vi "DAQmx Get Channel Property (CI Frequency Measurement Time).vi"(0 "task in":refnum<class "Session Factory.lvclass">, 11 "error in":errorcluster) -> (4 "task out":refnum<class "Session Factory.lvclass">, 6 "CI.Freq.MeasTime":dbl, 15 "error out":errorcluster)   [LabVIEW 2021, in "Session Management niDAQmx.lvlib" / "Session Factory.lvclass"]
doc: "<B>Property: Get DAQmx Channel (Counter Input:Frequency:Measurement Specifications:High Frequency:Measurement Time)</B>\n\nShort Name: <B>CI.Freq.MeasTime</B>\n\nSpecifies in seconds the length of time to measure the frequency of the signal if CI.Freq.MeasMeth is High Frequency with 2 Counters. Measurement accuracy increases with increased measurement time and with increased signal frequency. If you measure a high-frequency signal for too long, however, the count register could roll over, which results in an incorrect measurement."
uses:
  Session Factory.lvclass
  NI_DAQmx_client/RPC Messages/nidaqmx_grpc_GetChanAttributeDoubleRequest.ctl
  NI_DAQmx_client/RPC Messages/nidevice_grpc_Session.ctl
  NI_DAQmx_client/RPC Messages/nidevice_grpc_Session_session/nidevice_grpc_Session_session.lvclass
  NI_DAQmx_client/RPC Messages/nidaqmx_grpc_GetChanAttributeDoubleRequest_attribute_enum/nidaqmx_grpc_GetChanAttributeDoubleRequest_attribute_enum.lvclass
  NI_DAQmx_client/RPC Messages/nidaqmx_grpc_ChannelDoubleAttribute.ctl
  NI_DAQmx_client/RPC Messages/nidaqmx_grpc_GetChanAttributeDoubleRequest_attribute_enum/nidaqmx_grpc_GetChanAttributeDoubleRequest_attribute_enum.lvclass/nidaqmx_grpc_GetChanAttributeDoubleRequest_attribute_enum.ctl
  Session Factory.lvclass/Session Factory.ctl
  NI_DAQmx_client/NI_DAQmx_client.lvlib
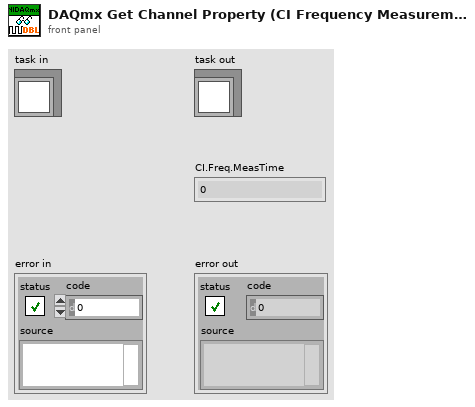
[diagram p1: front panel]
types:
  T1 = typedef "NI_DAQmx_client.lvlib/nidaqmx_grpc_ChannelDoubleAttribute.ctl" = enum32{"CHANNEL_DOUBLE_ATTRIBUTE_UNSPECIFIED", "CHANNEL_ATTRIBUTE_AI_IMPEDANCE", "CHANNEL_ATTRIBUTE_AI_AC_EXCIT_FREQ", "CHANNEL_ATTRIBUTE_AO_GAIN", "CHANNEL_ATTRIBUTE_AO_LOAD_IMPEDANCE", "CHANNEL_ATTRIBUTE_CI_FREQ_MEAS_TIME", "CHANNEL_ATTRIBUTE_CO_PULSE_FREQ_INITIAL_DELAY", "CHANNEL_ATTRIBUTE_AI_ACCEL_SENSITIVITY", "CHANNEL_ATTRIBUTE_AI_FREQ_HYST", "CHANNEL_ATTRIBUTE_AI_FREQ_THRESH_VOLTAGE", "CHANNEL_ATTRIBUTE_CI_ANG_ENCODER_INITIAL_ANGLE", "CHANNEL_ATTRIBUTE_CI_ENCODER_Z_INDEX_VAL", "CHANNEL_ATTRIBUTE_AI_RVDT_SENSITIVITY", "CHANNEL_ATTRIBUTE_CI_LIN_ENCODER_DIST_PER_PULSE", "CHANNEL_ATTRIBUTE_CI_LIN_ENCODER_INITIAL_POS", "CHANNEL_ATTRIBUTE_AI_LVDT_SENSITIVITY", "CHANNEL_ATTRIBUTE_AI_STRAIN_GAGE_GAGE_FACTOR", "CHANNEL_ATTRIBUTE_AI_STRAIN_GAGE_POISSON_RATIO", "CHANNEL_ATTRIBUTE_AI_RTD_A", "CHANNEL_ATTRIBUTE_AI_RTD_B", "CHANNEL_ATTRIBUTE_AI_RTD_C", "CHANNEL_ATTRIBUTE_AI_RTD_R0", "CHANNEL_ATTRIBUTE_AI_THRMCPL_CJC_VAL", "CHANNEL_ATTRIBUTE_AI_THRMSTR_R1", "CHANNEL_ATTRIBUTE_CO_PULSE_DUTY_CYC", "CHANNEL_ATTRIBUTE_CO_PULSE_FREQ", "CHANNEL_ATTRIBUTE_AO_MAX", "CHANNEL_ATTRIBUTE_AO_MIN", "CHANNEL_ATTRIBUTE_AO_OUTPUT_IMPEDANCE", "CHANNEL_ATTRIBUTE_AI_MICROPHONE_SENSITIVITY", "CHANNEL_ATTRIBUTE_AI_RESOLUTION", "CHANNEL_ATTRIBUTE_AI_MAX", "CHANNEL_ATTRIBUTE_AI_MIN", "CHANNEL_ATTRIBUTE_AI_BRIDGE_NOM_RESISTANCE", "CHANNEL_ATTRIBUTE_AI_BRIDGE_INITIAL_VOLTAGE", "CHANNEL_ATTRIBUTE_AI_LEAD_WIRE_RESISTANCE", "CHANNEL_ATTRIBUTE_AI_CURRENT_SHUNT_RESISTANCE", "CHANNEL_ATTRIBUTE_AI_EXCIT_VAL", "CHANNEL_ATTRIBUTE_AI_ATTEN", "CHANNEL_ATTRIBUTE_AI_LOWPASS_CUTOFF_FREQ", "CHANNEL_ATTRIBUTE_AI_HIGHPASS_CUTOFF_FREQ", "CHANNEL_ATTRIBUTE_AI_BANDPASS_CENTER_FREQ", "CHANNEL_ATTRIBUTE_AI_BANDPASS_WIDTH", "CHANNEL_ATTRIBUTE_AI_NOTCH_CENTER_FREQ", "CHANNEL_ATTRIBUTE_AI_NOTCH_WIDTH", "CHANNEL_ATTRIBUTE_AI_RNG_HIGH", "CHANNEL_ATTRIBUTE_AI_RNG_LOW", "CHANNEL_ATTRIBUTE_AI_GAIN", "CHANNEL_ATTRIBUTE_AO_RESOLUTION", "CHANNEL_ATTRIBUTE_AO_DAC_RNG_LOW", "CHANNEL_ATTRIBUTE_AO_DAC_RNG_HIGH", "CHANNEL_ATTRIBUTE_AO_DAC_REF_VAL", "CHANNEL_ATTRIBUTE_AI_EXCIT_ACTUAL_VAL", "CHANNEL_ATTRIBUTE_AI_LOWPASS_SWITCH_CAP_EXT_CLK_FREQ", "CHANNEL_ATTRIBUTE_CI_MAX", "CHANNEL_ATTRIBUTE_CI_MIN", "CHANNEL_ATTRIBUTE_CI_CTR_TIMEBASE_RATE", "CHANNEL_ATTRIBUTE_CO_PULSE_HIGH_TIME", "CHANNEL_ATTRIBUTE_CO_PULSE_LOW_TIME", "CHANNEL_ATTRIBUTE_CO_PULSE_TIME_INITIAL_DELAY", "CHANNEL_ATTRIBUTE_CO_CTR_TIMEBASE_RATE", "CHANNEL_ATTRIBUTE_AI_THRMSTR_A", "CHANNEL_ATTRIBUTE_AI_THRMSTR_C", "CHANNEL_ATTRIBUTE_AI_THRMSTR_B", "CHANNEL_ATTRIBUTE_CI_PERIOD_MEAS_TIME", "CHANNEL_ATTRIBUTE_AI_BRIDGE_SHUNT_CAL_GAIN_ADJUST", "CHANNEL_ATTRIBUTE_DI_DIG_FLTR_MIN_PULSE_WIDTH", "CHANNEL_ATTRIBUTE_CI_FREQ_DIG_FLTR_MIN_PULSE_WIDTH", "CHANNEL_ATTRIBUTE_CI_FREQ_DIG_FLTR_TIMEBASE_RATE", "CHANNEL_ATTRIBUTE_CI_PERIOD_DIG_FLTR_MIN_PULSE_WIDTH", "CHANNEL_ATTRIBUTE_CI_PERIOD_DIG_FLTR_TIMEBASE_RATE", "CHANNEL_ATTRIBUTE_CI_COUNT_EDGES_COUNT_DIR_DIG_FLTR_MIN_PULSE_WIDTH", "CHANNEL_ATTRIBUTE_CI_COUNT_EDGES_COUNT_DIR_DIG_FLTR_TIMEBASE_RATE", "CHANNEL_ATTRIBUTE_CI_COUNT_EDGES_DIG_FLTR_MIN_PULSE_WIDTH", "CHANNEL_ATTRIBUTE_CI_COUNT_EDGES_DIG_FLTR_TIMEBASE_RATE", "CHANNEL_ATTRIBUTE_CI_ENCODER_A_INPUT_DIG_FLTR_MIN_PULSE_WIDTH", "CHANNEL_ATTRIBUTE_CI_ENCODER_A_INPUT_DIG_FLTR_TIMEBASE_RATE", "CHANNEL_ATTRIBUTE_CI_ENCODER_B_INPUT_DIG_FLTR_MIN_PULSE_WIDTH", "CHANNEL_ATTRIBUTE_CI_ENCODER_B_INPUT_DIG_FLTR_TIMEBASE_RATE", "CHANNEL_ATTRIBUTE_CI_ENCODER_Z_INPUT_DIG_FLTR_MIN_PULSE_WIDTH", "CHANNEL_ATTRIBUTE_CI_ENCODER_Z_INPUT_DIG_FLTR_TIMEBASE_RATE", "CHANNEL_ATTRIBUTE_CI_PULSE_WIDTH_DIG_FLTR_MIN_PULSE_WIDTH", "CHANNEL_ATTRIBUTE_CI_PULSE_WIDTH_DIG_FLTR_TIMEBASE_RATE", "CHANNEL_ATTRIBUTE_CI_TWO_EDGE_SEP_FIRST_DIG_FLTR_MIN_PULSE_WIDTH", "CHANNEL_ATTRIBUTE_CI_TWO_EDGE_SEP_FIRST_DIG_FLTR_TIMEBASE_RATE", "CHANNEL_ATTRIBUTE_CI_TWO_EDGE_SEP_SECOND_DIG_FLTR_MIN_PULSE_WIDTH", "CHANNEL_ATTRIBUTE_CI_TWO_EDGE_SEP_SECOND_DIG_FLTR_TIMEBASE_RATE", "CHANNEL_ATTRIBUTE_CI_SEMI_PERIOD_DIG_FLTR_MIN_PULSE_WIDTH", "CHANNEL_ATTRIBUTE_CI_SEMI_PERIOD_DIG_FLTR_TIMEBASE_RATE", "CHANNEL_ATTRIBUTE_AI_SOUND_PRESSURE_MAX_SOUND_PRESSURE_LVL", "CHANNEL_ATTRIBUTE_AO_DAC_OFFSET_VAL", "CHANNEL_ATTRIBUTE_CI_CTR_TIMEBASE_DIG_FLTR_MIN_PULSE_WIDTH", "CHANNEL_ATTRIBUTE_CI_CTR_TIMEBASE_DIG_FLTR_TIMEBASE_RATE", "CHANNEL_ATTRIBUTE_CO_CTR_TIMEBASE_DIG_FLTR_MIN_PULSE_WIDTH", "CHANNEL_ATTRIBUTE_CO_CTR_TIMEBASE_DIG_FLTR_TIMEBASE_RATE", "CHANNEL_ATTRIBUTE_AI_VOLTAGE_DB_REF", "CHANNEL_ATTRIBUTE_AI_SOUND_PRESSURE_DB_REF", "CHANNEL_ATTRIBUTE_AI_ACCEL_DB_REF", "CHANNEL_ATTRIBUTE_AO_FUNC_GEN_FREQ", "CHANNEL_ATTRIBUTE_AO_FUNC_GEN_AMPLITUDE", "CHANNEL_ATTRIBUTE_AO_FUNC_GEN_OFFSET", "CHANNEL_ATTRIBUTE_AO_FUNC_GEN_SQUARE_DUTY_CYCLE", "CHANNEL_ATTRIBUTE_AO_VOLTAGE_CURRENT_LIMIT", "CHANNEL_ATTRIBUTE_AO_FUNC_GEN_FM_DEVIATION", "CHANNEL_ATTRIBUTE_DO_OVERCURRENT_LIMIT", "CHANNEL_ATTRIBUTE_DO_OVERCURRENT_REENABLE_PERIOD", "CHANNEL_ATTRIBUTE_AI_PROBE_ATTEN", "CHANNEL_ATTRIBUTE_AI_DC_OFFSET", "CHANNEL_ATTRIBUTE_AI_EDDY_CURRENT_PROX_PROBE_SENSITIVITY", "CHANNEL_ATTRIBUTE_DI_DIG_FLTR_TIMEBASE_RATE", "CHANNEL_ATTRIBUTE_CI_PULSE_FREQ_DIG_FLTR_MIN_PULSE_WIDTH", "CHANNEL_ATTRIBUTE_CI_PULSE_FREQ_DIG_FLTR_TIMEBASE_RATE", "CHANNEL_ATTRIBUTE_CI_PULSE_TIME_DIG_FLTR_MIN_PULSE_WIDTH", "CHANNEL_ATTRIBUTE_CI_PULSE_TIME_DIG_FLTR_TIMEBASE_RATE", "CHANNEL_ATTRIBUTE_CI_PULSE_TICKS_DIG_FLTR_MIN_PULSE_WIDTH", "CHANNEL_ATTRIBUTE_CI_PULSE_TICKS_DIG_FLTR_TIMEBASE_RATE", "CHANNEL_ATTRIBUTE_AI_BRIDGE_SHUNT_CAL_SHUNT_CAL_A_RESISTANCE", "CHANNEL_ATTRIBUTE_AI_BRIDGE_SHUNT_CAL_SHUNT_CAL_A_ACTUAL_RESISTANCE", "CHANNEL_ATTRIBUTE_AI_BRIDGE_SHUNT_CAL_SHUNT_CAL_B_RESISTANCE", "CHANNEL_ATTRIBUTE_AI_BRIDGE_SHUNT_CAL_SHUNT_CAL_B_ACTUAL_RESISTANCE", "CHANNEL_ATTRIBUTE_AI_FORCE_IEPE_SENSOR_SENSITIVITY", "CHANNEL_ATTRIBUTE_AI_BRIDGE_INITIAL_RATIO", "CHANNEL_ATTRIBUTE_AI_BRIDGE_TWO_POINT_LIN_FIRST_ELECTRICAL_VAL", "CHANNEL_ATTRIBUTE_AI_BRIDGE_TWO_POINT_LIN_FIRST_PHYSICAL_VAL", "CHANNEL_ATTRIBUTE_AI_BRIDGE_TWO_POINT_LIN_SECOND_ELECTRICAL_VAL", "CHANNEL_ATTRIBUTE_AI_BRIDGE_TWO_POINT_LIN_SECOND_PHYSICAL_VAL", "CHANNEL_ATTRIBUTE_CI_COUNT_EDGES_COUNT_RESET_DIG_FLTR_MIN_PULSE_WIDTH", "CHANNEL_ATTRIBUTE_CI_COUNT_EDGES_COUNT_RESET_DIG_FLTR_TIMEBASE_RATE", "CHANNEL_ATTRIBUTE_AI_THRMCPL_LEAD_OFFSET_VOLTAGE", "CHANNEL_ATTRIBUTE_AI_FILTER_DELAY", "CHANNEL_ATTRIBUTE_AI_VELOCITY_IEPE_SENSOR_DB_REF", "CHANNEL_ATTRIBUTE_AI_VELOCITY_IEPE_SENSOR_SENSITIVITY", "CHANNEL_ATTRIBUTE_AI_ROSETTE_STRAIN_GAGE_ORIENTATION", "CHANNEL_ATTRIBUTE_AO_FILTER_DELAY_ADJUSTMENT", "CHANNEL_ATTRIBUTE_AI_FILTER_DELAY_ADJUSTMENT", "CHANNEL_ATTRIBUTE_AO_FILTER_DELAY", "CHANNEL_ATTRIBUTE_CI_DUTY_CYCLE_DIG_FLTR_MIN_PULSE_WIDTH", "CHANNEL_ATTRIBUTE_CI_DUTY_CYCLE_DIG_FLTR_TIMEBASE_RATE", "CHANNEL_ATTRIBUTE_CI_MAX_MEAS_PERIOD", "CHANNEL_ATTRIBUTE_CI_THRESH_VOLTAGE", "CHANNEL_ATTRIBUTE_AI_DIG_FLTR_LOWPASS_CUTOFF_FREQ", "CHANNEL_ATTRIBUTE_AI_DIG_FLTR_HIGHPASS_CUTOFF_FREQ", "CHANNEL_ATTRIBUTE_AI_DIG_FLTR_BANDPASS_CENTER_FREQ", "CHANNEL_ATTRIBUTE_AI_DIG_FLTR_BANDPASS_WIDTH", "CHANNEL_ATTRIBUTE_AI_DIG_FLTR_NOTCH_CENTER_FREQ", "CHANNEL_ATTRIBUTE_AI_DIG_FLTR_NOTCH_WIDTH", "CHANNEL_ATTRIBUTE_CI_VELOCITY_LIN_ENCODER_DIST_PER_PULSE", "CHANNEL_ATTRIBUTE_CI_VELOCITY_ENCODER_A_INPUT_DIG_FLTR_MIN_PULSE_WIDTH", "CHANNEL_ATTRIBUTE_CI_VELOCITY_ENCODER_A_INPUT_DIG_FLTR_TIMEBASE_RATE", "CHANNEL_ATTRIBUTE_CI_VELOCITY_ENCODER_B_INPUT_DIG_FLTR_MIN_PULSE_WIDTH", "CHANNEL_ATTRIBUTE_CI_VELOCITY_ENCODER_B_INPUT_DIG_FLTR_TIMEBASE_RATE", "CHANNEL_ATTRIBUTE_CI_VELOCITY_MEAS_TIME", "CHANNEL_ATTRIBUTE_CI_COUNT_EDGES_GATE_DIG_FLTR_MIN_PULSE_WIDTH", "CHANNEL_ATTRIBUTE_CI_COUNT_EDGES_GATE_DIG_FLTR_TIMEBASE_RATE", "CHANNEL_ATTRIBUTE_AI_ACCEL_CHARGE_SENSITIVITY", "CHANNEL_ATTRIBUTE_AI_ACCEL_4_WIRE_DC_VOLTAGE_SENSITIVITY", "CHANNEL_ATTRIBUTE_AI_DATA_XFER_MAX_RATE", "CHANNEL_ATTRIBUTE_AI_SENSOR_POWER_VOLTAGE", "CHANNEL_ATTRIBUTE_AI_FILTER_FREQ", "CHANNEL_ATTRIBUTE_AI_INPUT_LIMITS_FAULT_DETECT_UPPER_LIMIT", "CHANNEL_ATTRIBUTE_AI_INPUT_LIMITS_FAULT_DETECT_LOWER_LIMIT", "CHANNEL_ATTRIBUTE_CI_FREQ_THRESH_VOLTAGE", "CHANNEL_ATTRIBUTE_CI_FREQ_HYST", "CHANNEL_ATTRIBUTE_CI_PERIOD_THRESH_VOLTAGE", "CHANNEL_ATTRIBUTE_CI_PERIOD_HYST", "CHANNEL_ATTRIBUTE_CI_COUNT_EDGES_THRESH_VOLTAGE", "CHANNEL_ATTRIBUTE_CI_COUNT_EDGES_HYST", "CHANNEL_ATTRIBUTE_CI_COUNT_EDGES_COUNT_DIR_THRESH_VOLTAGE", "CHANNEL_ATTRIBUTE_CI_COUNT_EDGES_COUNT_DIR_HYST", "CHANNEL_ATTRIBUTE_CI_COUNT_EDGES_COUNT_RESET_THRESH_VOLTAGE", "CHANNEL_ATTRIBUTE_CI_COUNT_EDGES_COUNT_RESET_HYST", "CHANNEL_ATTRIBUTE_CI_COUNT_EDGES_GATE_THRESH_VOLTAGE", "CHANNEL_ATTRIBUTE_CI_COUNT_EDGES_GATE_HYST", "CHANNEL_ATTRIBUTE_CI_FILTER_FREQ", "CHANNEL_ATTRIBUTE_CI_FILTER_DELAY", "CHANNEL_ATTRIBUTE_AO_FUNC_GEN_START_PHASE", "CHANNEL_ATTRIBUTE_AO_COMMON_MODE_OFFSET", "CHANNEL_ATTRIBUTE_PWR_VOLTAGE_SETPOINT", "CHANNEL_ATTRIBUTE_PWR_CURRENT_SETPOINT"}
  T2 = typedef "NI_DAQmx_client.lvlib/nidaqmx_grpc_GetChanAttributeDoubleRequest.ctl" = cluster{"task":T3, "channel":string, "nidaqmx_grpc_GetChanAttributeDoubleRequest_attribute_enum":refnum<class "nidaqmx_grpc_GetChanAttributeDoubleRequest_attribute_enum.lvclass">}
  T3 = typedef "NI_DAQmx_client.lvlib/nidevice_grpc_Session.ctl" = cluster{"nidevice_grpc_Session_session":refnum<class "nidevice_grpc_Session_session.lvclass">}
  T4 = typedef "grpc-lvsupport-release.lvlib/grpcId.ctl" = u64
  T5 = typedef "NI_DAQmx_client.lvlib/nidaqmx_grpc_GetChanAttributeDoubleResponse.ctl" = cluster{"status":i32, "value":dbl}
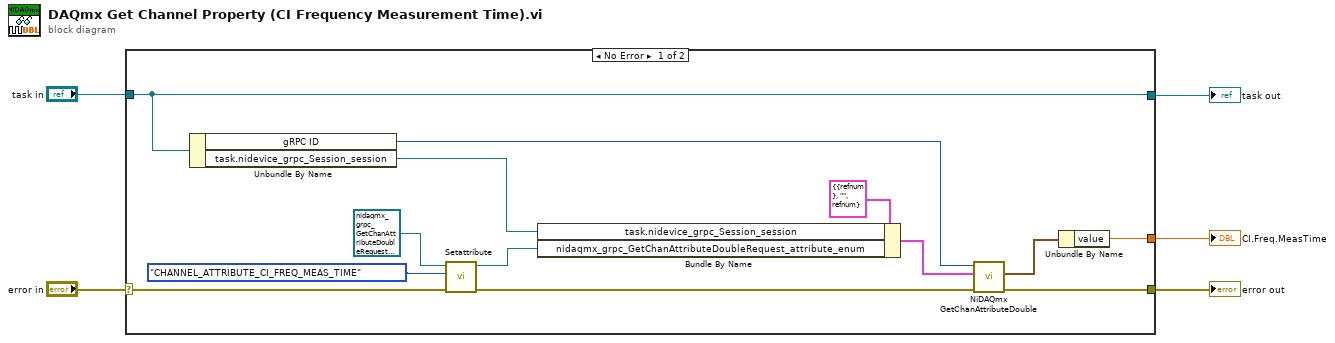
[diagram p0: block diagram]
diagram:
  n1 = case shown="No Error" "error in" {
    selector: "error in" -> [w12 w20]
    tunnel: [w16 w20] -> w4
    tunnel: "task in" -> [w17 w19]
    tunnel: [w17 w19] -> w2
    tunnel: [w6 _] -> w1
    frame No Error {
      n2 = Unbundle By Name(w17) -> ("gRPC ID"=w15:T4, "task.nidevice_grpc_Session_session"=w18:refnum<class "nidevice_grpc_Session_session.lvclass">)
      n3 = call "Setattribute.vi"("error in (no error)"=w12, "Set_Val"=nidaqmx_grpc_ChannelDoubleAttribute."CHANNEL_ATTRIBUTE_CI_FREQ_MEAS_TIME", "OneOfTemplate in"=refnum<class "nidaqmx_grpc_GetChanAttributeDoubleRequest_attribute_enum.lvclass"> refnum ("nidaqmx_grpc_GetChanAttributeDoubleRequest_attribute_enum")) -> ("error out"=w11:errorcluster, "OneOfTemplate out"=w9:refnum<class "nidaqmx_grpc_GetChanAttributeDoubleRequest_attribute_enum.lvclass">)  [unwired: 7 in]
      n4 = Bundle By Name(cluster=T2 {"task"={"nidevice_grpc_Session_session"=refnum}, "channel"="", "nidaqmx_grpc_GetChanAttributeDoubleRequest_attribute_enum"=refnum} ("Request Data"), "task.nidevice_grpc_Session_session"=w18, "nidaqmx_grpc_GetChanAttributeDoubleRequest_attribute_enum"=w9) -> (w8:T2)
      n5 = call "NiDAQmx GetChanAttributeDouble.vi"("error in"=w11, "Request Data"=w8, "gRPC ID"=w15) -> ("error out"=w16:errorcluster, "Response Data"=w7:T5)  [unwired: 6 in, 1 out]
      n6 = Unbundle By Name(w7) -> ("value"=w6:dbl)
    }
    frame Error {
    }
  }
  "error out" <- w4
  "task out" <- w2
  "CI.Freq.MeasTime" <- w1
